vi "Insert.vi"(6 "Item":T1={"Item offset"=0, "Offset past Item"=0, "Name offset"=0, "Offset past Name"=0, "Found"=FALSE, "Item Type"=enum."Parser Error", "Item Index"=-1, "Start Offset"=-1, "Comma Needed For Insert"=FALSE}, 9 "<JSON>name":string, 10 "JSON to Insert":string, 11 "JSON in":string) -> (1 "Inserted Item Offset":i32, 2 "Found":bool, 3 "string":string)   [LabVIEW 2019, in "JSONtext.lvlib"]
uses:
  JSONtext.lvlib
  Parsing/Found Items.ctl
  Parsing/Parsing State.ctl
  Parsing/Advance past replacable whitespace.vi
  JDP Science Common Utilities/Trim Whitespace__JDP.vi
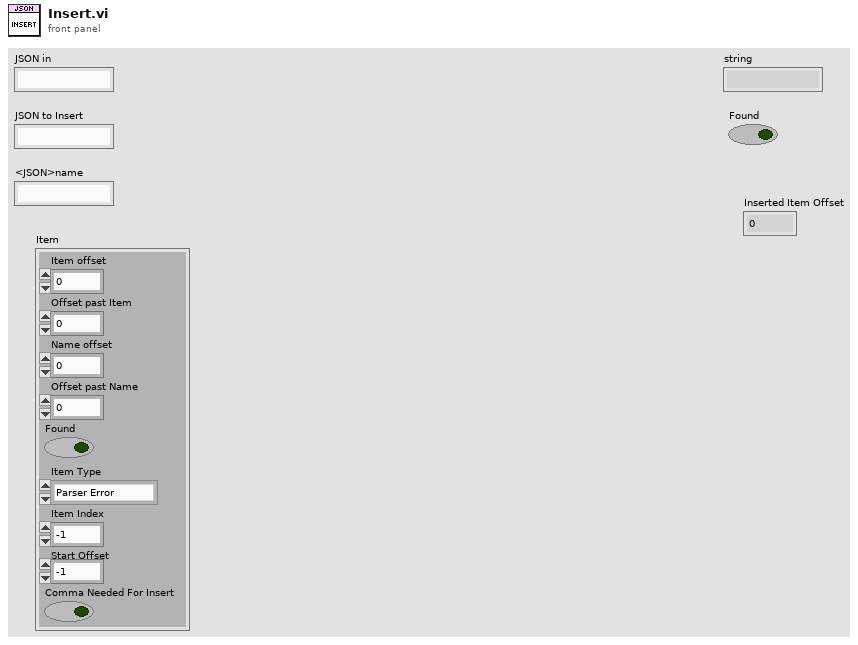
[diagram p1: front panel]
types:
  T1 = typedef "JSONtext.lvlib/Found Items.ctl" = cluster{"Item offset":i32, "Offset past Item":i32, "Name offset":i32, "Offset past Name":i32, "Found":bool, "Item Type":T2, "Item Index":i32, "Start Offset":i32, "Comma Needed For Insert":bool}
  T2 = typedef "JSONtext.lvlib/Parsing State.ctl" = enum16{"Parser Error", "Object", "Array", "String", "Number/Other", "Leading Whitespace", "Object end", "Array end", "Value end"}
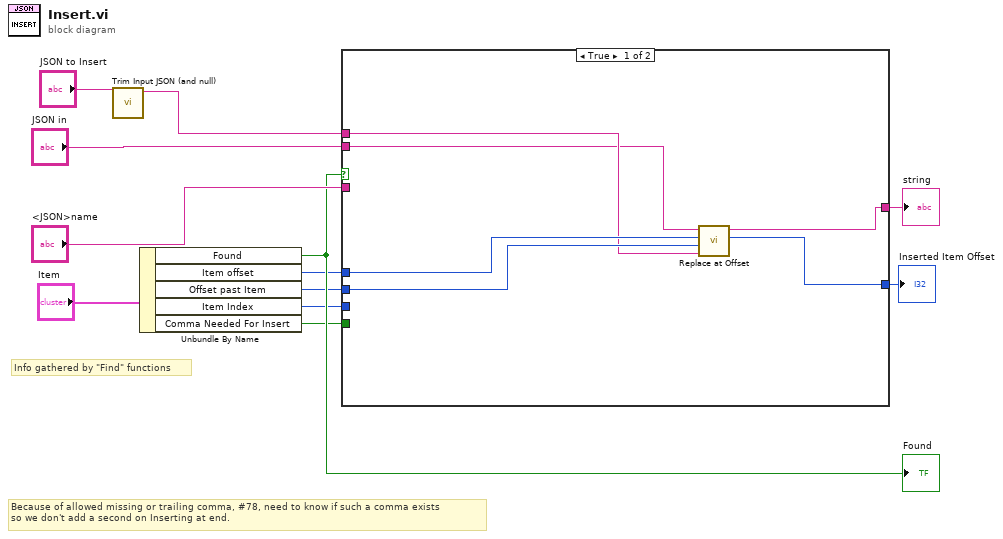
[diagram p0: block diagram]
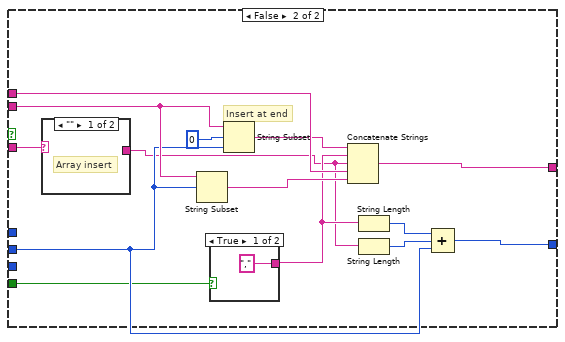
[diagram p2: hidden frame]
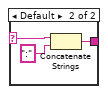
[diagram p3: hidden frame]
diagram:
  # "Info gathered by \"Find\" functions"
  # "Because of allowed missing or trailing comma, #78, need to know if such a comma exists \nso we don't add a second on Inserting at end."
  n1 = call "Trim Input JSON (and null).vi"("JSON Input"="JSON to Insert") -> ("<JSON>"=w2:string)  [unwired: 10 in]
  n2 = Unbundle By Name("Item") -> ("Found"=w11:bool, "Item offset"=w8:i32, "Offset past Item"=w7:i32, "Item Index"=w6:i32, "Comma Needed For Insert"=w1:bool)
  "Found" <- w11
  n3 = case shown="True" w11 {
    tunnel: "JSON in" -> [w14 w32]
    tunnel: w2 -> [w15 w31]
    tunnel: [w18 w30] -> w9
    tunnel: "<JSON>name" -> [_ w21]
    tunnel: w8 -> [w17 _]
    tunnel: w7 -> [w16 w22]
    tunnel: w6 -> [_ _]
    tunnel: [w13 w23] -> w4
    tunnel: w1 -> [_ w19]
    frame True {
      n4 = call "Replace at Offset.vi"("JSON to Insert"=w15, "Offset past Item"=w16, "Item offset"=w17, "<JSON> in"=w14) -> ("Item offset"=w13:i32, "<JSON>"=w18:string)  [unwired: 6 in]
    }
    frame False {
      # "Insert at end"
      n5 = case shown="\"\"" w21 {
        selector: w21 -> [_ w34]
        tunnel: [_ w33] -> w20
        frame "" {
          # "Array insert"
        }
        frame Default {
          n6 = Concatenate Strings(w34, ":" ("string")) -> (w33:string)
        }
      }
      n7 = String Subset(string=w32, offset (0)=w22) -> (substring=w27:string)  [unwired: 1 in]
      n8 = case shown="True" w19 {
        tunnel: ["," ("string") _] -> w26
        frame True {
        }
        frame False {
        }
      }
      n9 = String Subset(string=w32, offset (0)=0 ("Value start in"), length (rest)=w22) -> (substring=w28:string)
      n10 = Concatenate Strings(w28, w26, w20, w31, w27) -> (w30:string)
      n11 = String Length(string=w26) -> (length=w25:i32)
      n12 = String Length(string=w20) -> (length=w24:i32)
      n13 = Compound Arithmetic op=ADD(w25, w24, w22) -> (w23:i32)
    }
  }
  "string" <- w9
  "Inserted Item Offset" <- w4
